vi "Elevator Controller.vi"(8 "error in (no error)":errorcluster, 9 "Variables":T1, 10 "User Events":T10, 11 "Queues":T11) -> (0 "error out":errorcluster)   [LabVIEW 2017]
uses:
  support/Controls/User Events.ctl
  Error Handler/Controls/Error EventData.ctl
  Error Handler/Controls/Error Type.ctl
  support/Message Queue/All Message Queues.ctl
  support/Message Queue/Message Cluster.ctl
  Configuration/Controls/Config Commands.ctl
  Configuration/Controls/ConfigStates.ctl
  Controls/Elevator Command Event.ctl
  Controls/Elevator Commands.ctl
  support/Controls/Shared Variables.ctl
  Configuration/Controls/ConfigData.ctl
  Controls/Elevator Overhead.ctl
  Controls/Elevator States.ctl
  Controls/Elevator Location.ctl
  support/User Events/User Events.lvlib
  support/Message Queue/Message Queue.lvlib
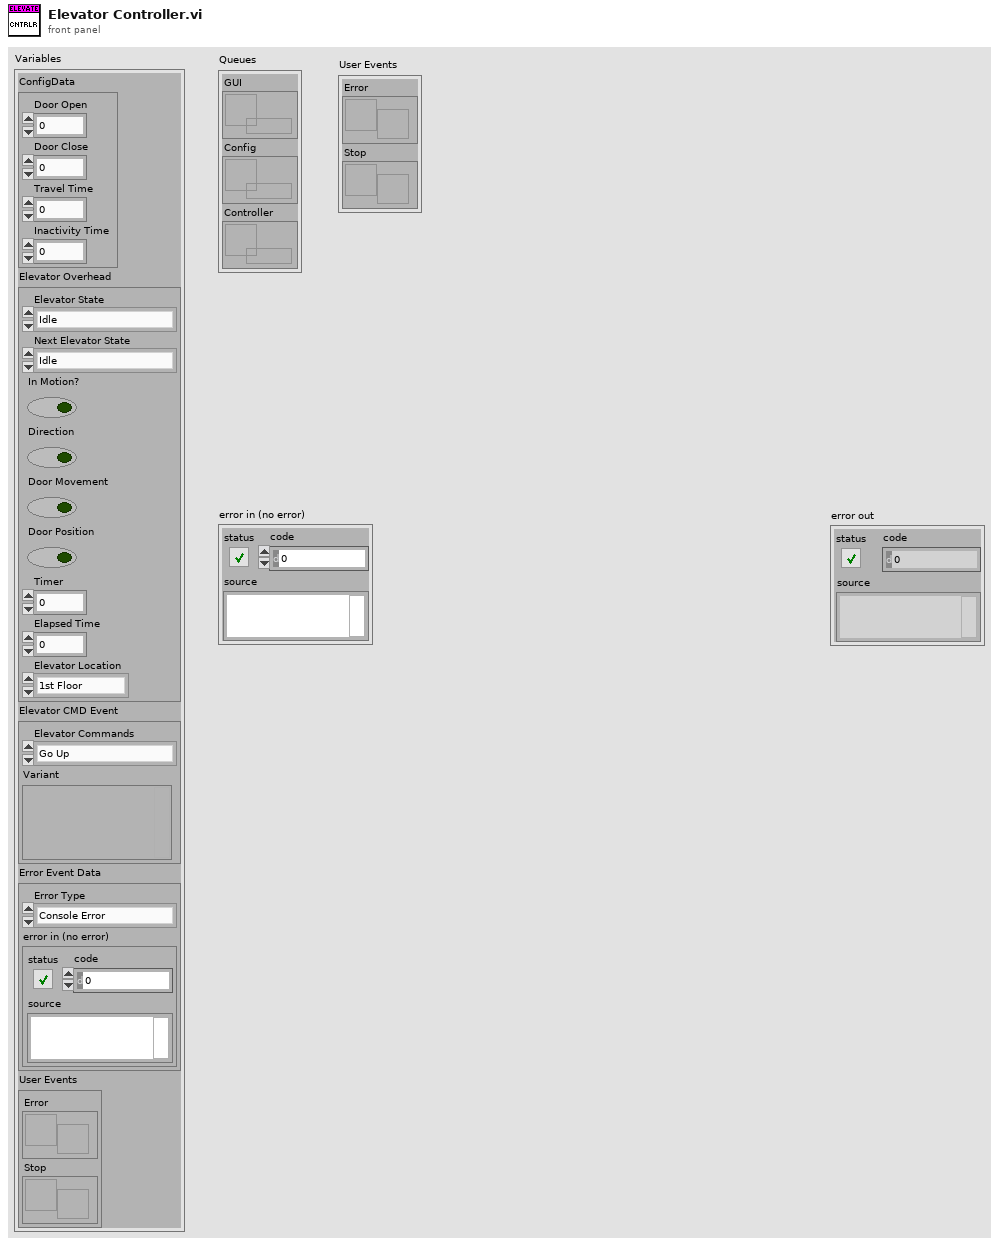
[diagram p1: front panel]
types:
  T1 = typedef "Shared Variables.ctl" = cluster{"ConfigData":T2, "Elevator Overhead":T3, "Elevator CMD Event":T6, "Error Event Data":T8, "User Events":T10}
  T2 = typedef "ConfigData.ctl" = cluster{"Door Open":dbl, "Door Close":dbl, "Travel Time":dbl, "Inactivity Time":dbl}
  T3 = typedef "Elevator Overhead.ctl" = cluster{"Elevator State":T4, "Next Elevator State":T4, "In Motion?":bool, "Direction":bool, "Door Movement":bool, "Door Position":bool, "Timer":dbl, "Elapsed Time":dbl, "Elevator Location":T5}
  T4 = typedef "Elevator States.ctl" = enum16{"Idle", "Init", "Open Doors", "Close Doors", "Start Move", "Move", "Finish Move", "Analysis", "Emergency"}
  T5 = typedef "Elevator Location.ctl" = enum16{"1st Floor", "2nd Floor", "3rd Floor", "4th Floor"}
  T6 = typedef "Elevator Command Event.ctl" = cluster{"Elevator Commands":T7, "Variant":variant}
  T7 = typedef "Elevator Commands.ctl" = enum16{"Go Up", "Go Down", "Go to Floor", "Emergency", "Open Doors", "Close Doors", "Start Move", "Move", "Finish Move", "Analysis", "Init", "Shutdown"}
  T8 = typedef "Error EventData.ctl" = cluster{"Error Type":T9, "error in (no error)":errorcluster}
  T9 = typedef "Error Type.ctl" = enum16{"Console Error", "Sensor Interface IO Error", "Process Step Error"}
  T10 = typedef "User Events.ctl" = cluster{"Error":refnum<user-event>, "Stop":refnum<user-event>}
  T11 = typedef "Message Queue.lvlib/All Message Queues.ctl" = cluster{"GUI":refnum<queue>, "Config":refnum<queue>, "Controller":refnum<queue>}
  T12 = typedef "Message Queue.lvlib/Message Cluster.ctl" = cluster{"Message":string, "Message Data":variant}
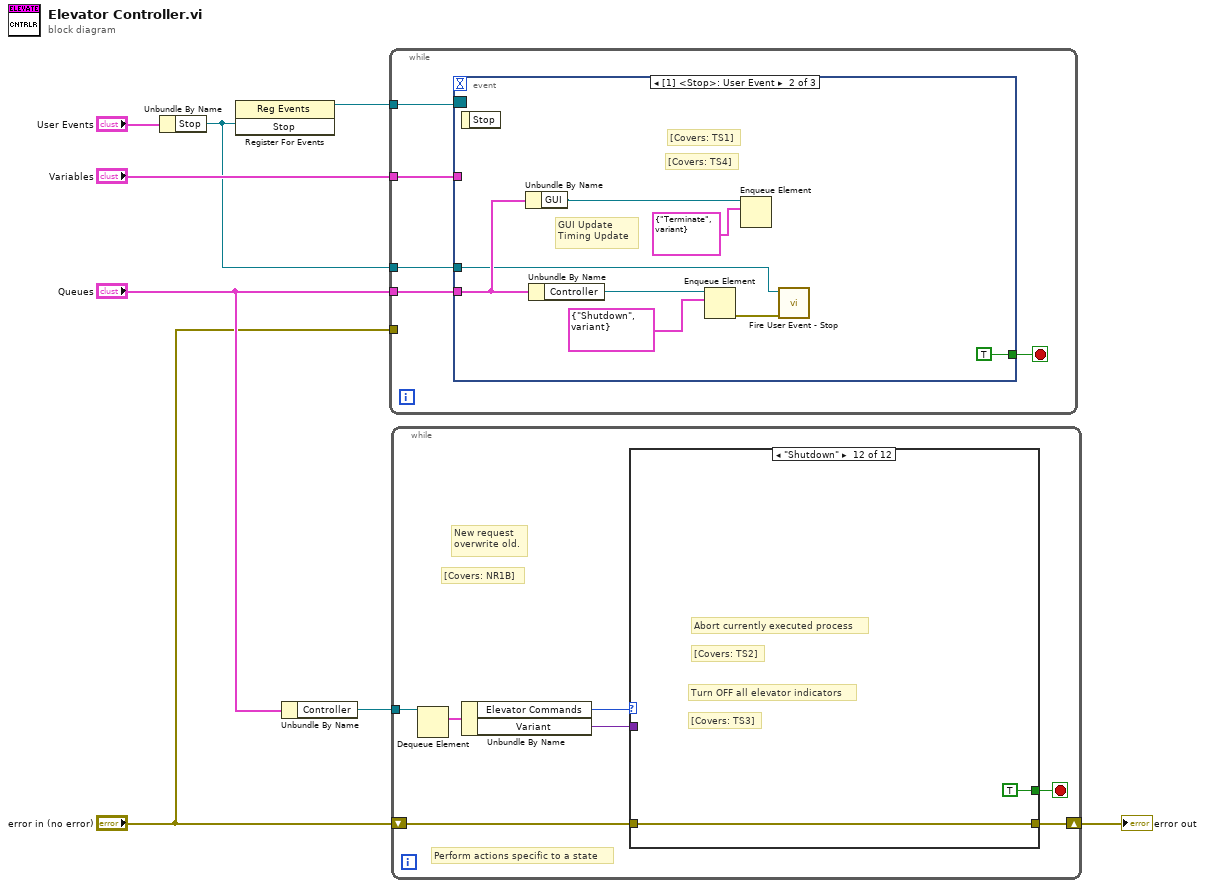
[diagram p0: block diagram]
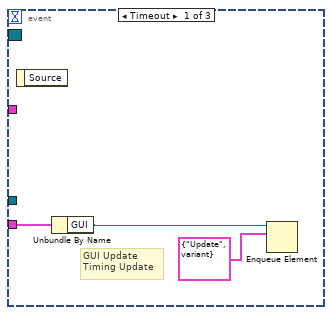
[diagram p13: hidden frame]
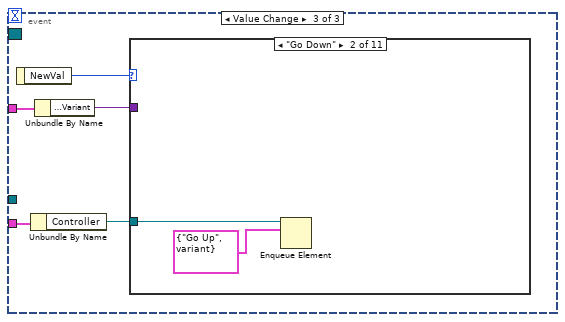
[diagram p14: hidden frame]
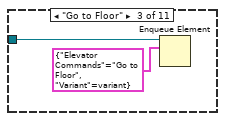
[diagram p16: hidden frame]
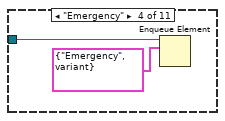
[diagram p17: hidden frame]
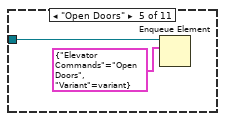
[diagram p18: hidden frame]
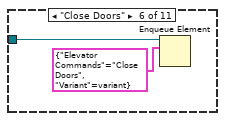
[diagram p19: hidden frame]
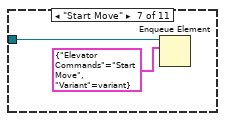
[diagram p20: hidden frame]
diagram:
  n1 = Unbundle By Name("User Events") -> ("Stop"=w1:refnum<user-event>)
  n2 = register-events(w1) -> (reference out=w7:refnum<event-registration>)  [unwired: 2 in, 1 out]
  n3 = Unbundle By Name("Queues") -> ("Controller"=w4:refnum<queue>)
  n4 = while {
    tunnel: w7 -> [w13]
    tunnel: "Queues" -> [w11]
    tunnel: "Variables" -> [w10]
    tunnel: "error in (no error)" -> [_]
    tunnel: w1 -> [w9]
    stop <- w12 stop-if-true
    n5 = event shown="[1] <Stop>: User Event" {
      selector: w13 -> [_ _ _]
      dyn-events: _ -> [_ _ _]
      timeout: _ -> [_ _ _]
      tunnel: [_ TRUE _] -> w12
      tunnel: w11 -> [w16 w18 w26]
      tunnel: w10 -> [_ _ w29]
      tunnel: w9 -> [_ w17 _]
      event Timeout {
        # "GUI Update\nTiming Update"
        n6 = event-data() -> ()  [unwired: 1 in, 1 out]
        n7 = Unbundle By Name(w16) -> ("GUI"=w15:refnum<queue>)
        n8 = Enqueue Element(queue=w15, element=T12 {"Message"="Update", "Message Data"=variant}) -> ()  [unwired: 2 in, 3 out]
      }
      event User Event {
        # "[Covers: TS1]"
        # "[Covers: TS4]"
        # "GUI Update\nTiming Update"
        n9 = event-data() -> ()  [unwired: 1 in, 1 out]
        n10 = Unbundle By Name(w18) -> ("GUI"=w20:refnum<queue>)
        n11 = Unbundle By Name(w18) -> ("Controller"=w22:refnum<queue>)
        n12 = Enqueue Element(queue=w22, element=T6 {"Elevator Commands"=enum."Shutdown", "Variant"=variant} ("Elevator CMD Event")) -> (error out=w21:errorcluster)  [unwired: 2 in, 2 out]
        n13 = Enqueue Element(queue=w20, element=T12 {"Message"="Terminate", "Message Data"=variant}) -> ()  [unwired: 2 in, 3 out]
        n14 = call "Fire User Event - Stop.vi"("error in (no error)"=w21, "User Event - Stop"=w17) -> ()  [unwired: 9 in, 1 out]
      }
      event Value Change {
        n15 = event-data() -> ("NewVal"=w28:T7)  [unwired: 1 in]
        n16 = Unbundle By Name(w26) -> ("Controller"=w25:refnum<queue>)
        n17 = Unbundle By Name(w29) -> ("Elevator CMD Event.Variant"=w27:variant)
        n18 = case shown="\"Go Down\"" w28 {
          tunnel: w27 -> [_ _ _ _ _ _ _ _ _ _ _]
          tunnel: w25 -> [_ w30 w32 w34 w36 w38 w40 w42 w44 w46 w48]
          frame Default {
          }
          frame "Go Down" {
            n19 = Enqueue Element(queue=w30, element=T6 {"Elevator Commands"=enum."Go Up", "Variant"=variant} ("Elevator CMD Event")) -> ()  [unwired: 2 in, 3 out]
          }
          frame "Go to Floor" {
            n20 = Enqueue Element(queue=w32, element=T6 {"Elevator Commands"=enum."Go to Floor", "Variant"=variant} ("Elevator CMD Event")) -> ()  [unwired: 2 in, 3 out]
          }
          frame "Emergency" {
            n21 = Enqueue Element(queue=w34, element=T6 {"Elevator Commands"=enum."Emergency", "Variant"=variant} ("Elevator CMD Event")) -> ()  [unwired: 2 in, 3 out]
          }
          frame "Open Doors" {
            n22 = Enqueue Element(queue=w36, element=T6 {"Elevator Commands"=enum."Open Doors", "Variant"=variant} ("Elevator CMD Event")) -> ()  [unwired: 2 in, 3 out]
          }
          frame "Close Doors" {
            n23 = Enqueue Element(queue=w38, element=T6 {"Elevator Commands"=enum."Close Doors", "Variant"=variant} ("Elevator CMD Event")) -> ()  [unwired: 2 in, 3 out]
          }
          frame "Start Move" {
            n24 = Enqueue Element(queue=w40, element=T6 {"Elevator Commands"=enum."Start Move", "Variant"=variant} ("Elevator CMD Event")) -> ()  [unwired: 2 in, 3 out]
          }
          frame "Move" {
            n25 = Enqueue Element(queue=w42, element=T6 {"Elevator Commands"=enum."Move", "Variant"=variant} ("Elevator CMD Event")) -> ()  [unwired: 2 in, 3 out]
          }
          frame "Finish Move" {
            n26 = Enqueue Element(queue=w44, element=T6 {"Elevator Commands"=enum."Finish Move", "Variant"=variant} ("Elevator CMD Event")) -> ()  [unwired: 2 in, 3 out]
          }
          frame "Analysis" {
            n27 = Enqueue Element(queue=w46, element=T6 {"Elevator Commands"=enum."Analysis", "Variant"=variant} ("Elevator CMD Event")) -> ()  [unwired: 2 in, 3 out]
          }
          frame "Go Up" {
            n28 = Enqueue Element(queue=w48, element=T6 {"Elevator Commands"=enum."Go Up", "Variant"=variant} ("Elevator CMD Event")) -> ()  [unwired: 2 in, 3 out]
          }
        }
      }
    }
  }
  n29 = while {
    tunnel: w4 -> [w56]
    shift-right: [w51] -> w3
    shift-left: "error in (no error)" -> [w52]
    stop <- w50 stop-if-true
    # "Perform actions specific to a state"
    # "[Covers: NR1B]"
    # "New request \noverwrite old."
    n30 = Dequeue Element(queue=w56) -> (element=w55:T6)  [unwired: 2 in, 3 out]
    n31 = Unbundle By Name(w55) -> ("Elevator Commands"=w54:T7, "Variant"=w53:variant)
    n32 = case shown="\"Shutdown\"" w54 {
      tunnel: w53 -> [_ _ _ _ _ _ _ _ _ _ _ _]
      tunnel: w52 -> [w57 w58 w59 w60 w61 w62 w63 w64 w65 w66 w67 w69]
      tunnel: [w57 w58 w59 w60 w61 w62 w63 w64 w65 w66 w67 w69] -> w51
      tunnel: [_ _ _ _ _ _ _ _ _ _ _ TRUE] -> w50
      frame "Go Up", Default {
        # "[Covers: OC3A]"
        # "Go to elevator move up state\nby setting next state in View Model"
      }
      frame "Go Down" {
        # "Go to elevator move down state\nby setting next state in View Model"
      }
      frame "Go to Floor" {
        # "[Covers: WS3]"
        # "[Covers: WS2]"
        # "If on the first floor, set open doors to next state,\nelse set travel state"
        # "Go to elevator move up/down state\nby setting next state in View Model"
      }
      frame "Emergency" {
        # "Go to elevator emergency state\nby setting next state in View Model"
      }
      frame "Open Doors" {
        # "[Covers: OC3B]"
        # "If open door timer <=0, go to close state"
        # "[Covers: SS1]"
        # "Send digital output to open doors. Fire door open event"
        # "[Covers: OC3A]"
        # "[Covers: OC3]"
        # "Start open door timer"
        # "Go to elevator open doors state\nby setting next state in View Model"
      }
      frame "Close Doors" {
        # "[Covers: OC7]"
        # "Transition to initial state"
        # "Go to elevator close doors state\nby setting next state in View Model"
      }
      frame "Start Move" {
        # "[Covers: OC6]"
        # "Fire a motion event"
        # "[Covers: CT1]"
        # "[Covers: SS4]"
        # "Initialize travel timer in view model"
      }
      frame "Move" {
        # "[Covers: CT1B]"
        # "[Covers: SS4B]"
        # "If time has elapsed, stop elevator. Update floor position"
        # "[Covers: CT1A]"
        # "[Covers: SS4A]"
        # "Update elapsed time and elevator location"
      }
      frame "Finish Move" {
        # "[Covers: RF3]"
        # "Transition to door open/close"
      }
      frame "Analysis" {
        # "[Covers: AS2C]"
        # "[Covers: AS2B]"
        # "[Covers: AS2A]"
        # "[Covers: AS2]"
        # "[Covers: AS1]"
        # "Handles all analysis"
      }
      frame "Init" {
        # "[Covers: NR1A]"
        # "If inactivity timer <=0, transition to start move with 1st floor as destination"
        # "[Covers: NR1]"
        # "Countdown inactivity timer to zero if >0."
        # "[Covers: WS1]"
        # "Maintain initial state defaults"
      }
      frame "Shutdown" {
        # "[Covers: TS3]"
        # "Turn OFF all elevator indicators"
        # "[Covers: TS2]"
        # "Abort currently executed process"
      }
    }
  }
  "error out" <- w3
